vi "Obtain-PAQ-Queue.vi"() -> (6 "queue out":refnum<queue>)   [LabVIEW 2014, in "HISW.lvclass"]
doc: "Obtain a queue for PAQ acquisition"
uses:
  HISW.lvclass
  controls/typedef_PAQsample.ctl
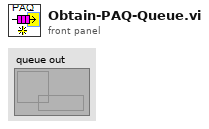
[diagram p1: front panel]
types:
  T1 = typedef "typedef_PAQsample.ctl" = cluster{"Time Stamp":timestamp, "TAGs":string[], "status":u32[], "data":dbl[], "Source":string}
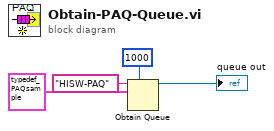
[diagram p0: block diagram]
diagram:
  n1 = Obtain Queue(max queue size (-1, unlimited)=1000, name (unnamed)="HISW-PAQ", element data type=T1 {"Time Stamp"=timestamp(0 s since 1904-01-01), "TAGs"=[], "status"=[], "data"=[], "Source"=""} ("DAQ")) -> (queue out=→"queue out":refnum<queue>)  [unwired: 2 in, 2 out]
